vi "readRateHtml.vi"(7 "Web(T)":bool=TRUE, 8 "Error In":errorcluster, 11 "url":string="http://195.77.159.50:8008/rate.txt") -> (0 "Error Out":errorcluster, 1 "Hora":string="17:44", 2 "Fecha":string="25/05/1951", 3 "datoNuevo?":bool=TRUE, 4 "datosGraficaRateNum":T1 {"FreqRun" format="%.1f"; "Frequency" format="%.1f"; "Time" format="%.1f"; "TotalBlocks" format="%.1f"; "Block" format="%.1f"}, 5 "Fecha":string="1495730694", 6 "datosGraficaRate":T2)   [LabVIEW 2013]
uses:
  datosGraficaRateString.ctl
  datosGraficaRateNumeric.ctl
  <vilib>/httpClient/LabVIEWHTTPClient.lvlib
panel:
  out "Array Date":string[](array[string])
  out "after substring":string
  out "Array":string[](array[string])
  out "body":string="1495730694 0,000000 1100,000000 1050,250000 985,000000 885,750000 901,500000 970,500000 900,500000 823,500000 1049,500000 913,250000 1013,250000 0,000000 927,500000 949,250000 1025,500000 1000,750000 905,500000 1050,250000 950,750000 0,250000 0,250000 0,000000 0,001000\r\n"
  out "headers":string="HTTP/1.1 200 OK\r\nDate: Wed, 31 May 2017 21:19:10 GMT\r\nServer: Apache/2.4.25 (Win32) OpenSSL/1.0.2j PHP/7.1.4\r\nLast-Modified: Tue, 30 May 2017 21:29:51 GMT\r\nETag: \"10f-550c480f7c17c\"\r\nAccept-Ranges: bytes\r\nContent-Length: 271\r\nContent-Type: text/plain\r\n\r\n"
  # "LEE EL FICHERO TXT ALMACENADO EN EL SERVIDOR WEB\nEXTRAE LOS VALORES ORDENADOS A UNA MATRIZ"
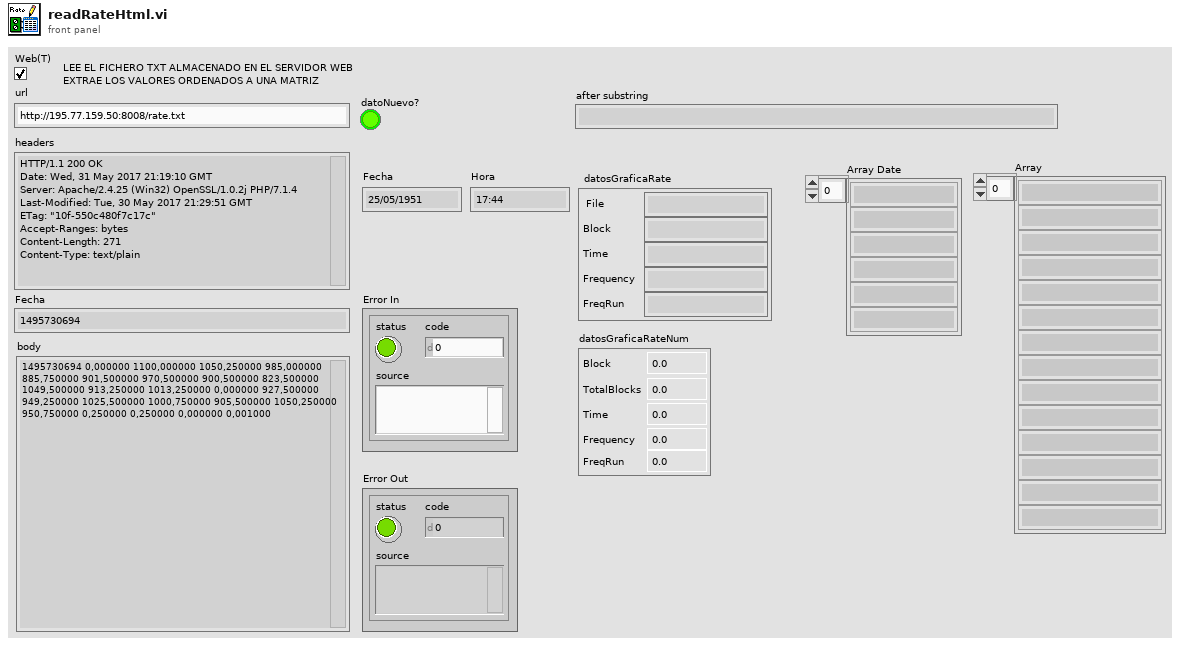
[diagram p1: front panel]
types:
  T1 = typedef "datosGraficaRateNumeric.ctl" = cluster{"Block":dbl, "TotalBlocks":dbl, "Time":dbl, "Frequency":dbl, "FreqRun":dbl}
  T2 = typedef "datosGraficaRateString.ctl" = cluster{" File":string, "Block":string, "Time":string, "Frequency":string, "FreqRun":string}
  T3 = typedef "LabVIEWHTTPClient.lvlib/ClientHandle.ctl" = refnum<k1>
  T4 = cluster{"[0]":string, "[1]":string, "[2]":string, "[3]":string, "[4]":string}
  T5 = cluster{"[0]":dbl, "[1]":dbl, "[2]":dbl, "[3]":dbl, "[4]":dbl}
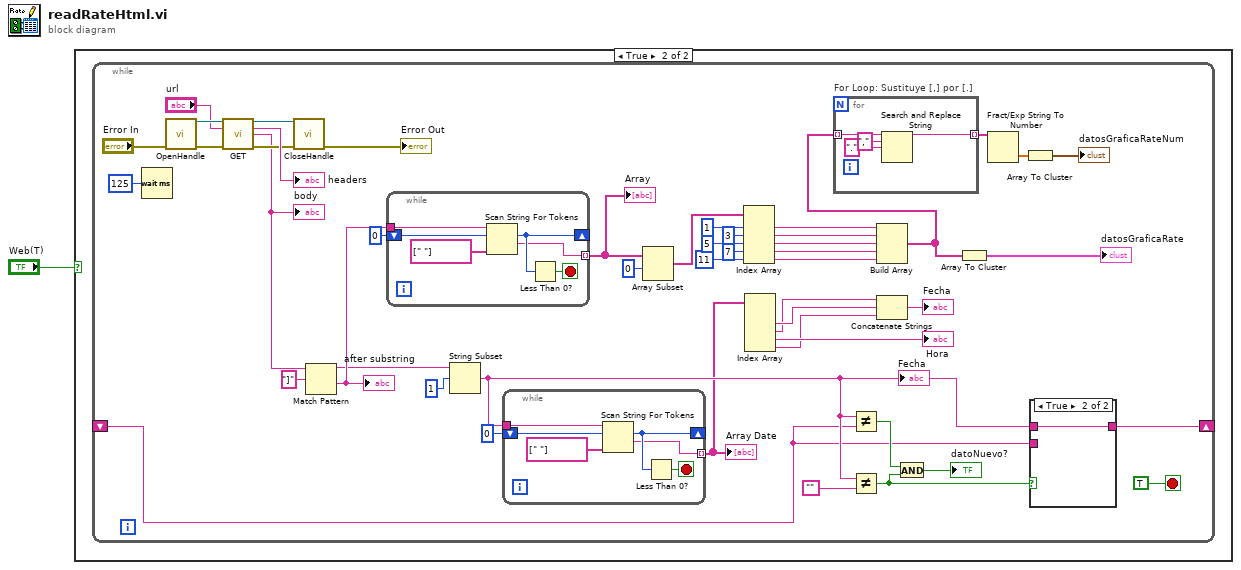
[diagram p0: block diagram]
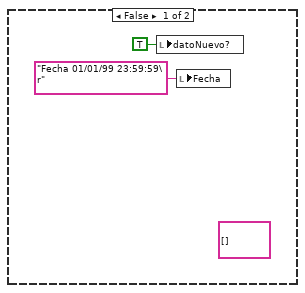
[diagram p2: hidden frame]
diagram:
  n1 = case shown="True" "Web(T)" {
    frame False {
      (unwired) string[][] []
      n2 = local write "datoNuevo?"(TRUE ("datoNuevo?")) -> ()
      n3 = local write "Fecha"("Fecha 01/01/99 23:59:59\r" ("Fecha")) -> ()
    }
    frame True {
      n4 = while {
        shift-right: [w36] -> _
        shift-left: _ -> [w11]
        stop <- TRUE stop-if-true
        n5 = Wait (ms)(milliseconds to wait=u32 125) -> ()  [unwired: 1 out]
        n6 = call <vilib>:"OpenHandle.vi"("error in (no error)"="Error In") -> ("client handle out"=w51:T3, "error out"=w47:errorcluster)  [unwired: 13 in]
        n7 = call <vilib>:"GET.vi"("client handle"=w51, "url"="url", "error in (no error)"=w47) -> ("client handle out"=w50:T3, "headers"=→"headers":string, "body"=w16:string, "error out"=w48:errorcluster)  [unwired: 9 in]
        "body" <- w16
        n8 = call <vilib>:"CloseHandle.vi"("client handle"=w50, "error in (no error)"=w48) -> ("error out"=→"Error Out":errorcluster)  [unwired: 13 in]
        n9 = Match Pattern(string=w16, regular expression="]") -> (before substring=w14:string, after substring=w15:string)  [unwired: 1 in, 2 out]
        "after substring" <- w15
        n10 = while {
          tunnel: w15 -> [w69]
          shift-right: [w65] -> _
          shift-left: 0 ("offset past token") -> [w67]
          tunnel: [w64] -> w42 mode=indexing
          stop <- w66 stop-if-true
          n11 = Scan String For Tokens(6:string[] [" "] ("delimiters (\\s,\\t,\\r,\\n)"), 8:w67, 9:w69) -> (1:w64:string, 2:w65:i32)  [unwired: 3 in, 2 out]
          n12 = Less Than 0?(x=w65) -> (x < 0?=w66:bool)
        }
        "Array" <- w42
        n13 = String Subset(string=w14, offset (0)=1 ("length (rest)")) -> (substring=w12:string)  [unwired: 1 in]
        "Fecha" <- w12
        n14 = while {
          tunnel: w12 -> [w57]
          shift-right: [w53] -> _
          shift-left: 0 ("offset past token") -> [w55]
          tunnel: [w52] -> w10 mode=indexing
          stop <- w54 stop-if-true
          n15 = Scan String For Tokens(6:string[] [" "] ("delimiters (\\s,\\t,\\r,\\n)"), 8:w55, 9:w57) -> (1:w52:string, 2:w53:i32)  [unwired: 3 in, 2 out]
          n16 = Less Than 0?(x=w53) -> (x < 0?=w54:bool)
        }
        "Array Date" <- w10
        n17 = Array Subset(array=w42, index=0) -> (w32:string[])  [unwired: 1 in]
        n18 = Index Array(array=w32, index #1=1 ("index"), index #2=3 ("index"), index #3=5 ("index"), index #4=7 ("index"), index #5=11 ("index")) -> (element #1=w33:string, element #2=w31:string, element #3=w30:string, element #4=w29:string, element #5=w28:string)
        n19 = Index Array(array=w10) -> (element #2=w6:string, element #3=w5:string, element #4=→"Hora":string, element #5=w8:string)  [unwired: 5 in, 1 out]
        n20 = Not Equal?(x=w12, y=w11) -> (x != y?=w39:bool)
        n21 = Not Equal?(x=w12, y="") -> (x != y?=w37:bool)
        n22 = Build Array(w33, w31, w30, w29, w28) -> (w20:string[])
        n23 = for "For Loop: Sustituye [,] por [.]" {
          tunnel: w20 -> [w61] mode=indexing
          tunnel: [w58] -> w22 mode=indexing
          n24 = Search and Replace String(input string=w61, search string=",", replace string="." ("replace string (\"\")")) -> (result string=w58:string)  [unwired: 5 in, 3 out]
        }
        n25 = Concatenate Strings(w5, w6, w8) -> (→"Fecha":string)
        n26 = And(x=w39, y=w37) -> (x .and. y?=→"datoNuevo?":bool)
        n27 = Array To Cluster(array=w20) -> (cluster=→"datosGraficaRate":T4)
        n28 = Fract/Exp String To Number(string=w22) -> (number=w21:dbl[])  [unwired: 3 in, 1 out]
        n29 = Array To Cluster(array=w21) -> (cluster=→"datosGraficaRateNum":T5)
        n30 = case shown="True" w37 {
          tunnel: w12 -> [_ w63]
          tunnel: [w62 w63] -> w36
          tunnel: w11 -> [w62 _]
          frame False {
          }
          frame True {
          }
        }
      }
    }
  }
